vi "Watchdog Extended.vi"(11 "Enable Watchdog":bool=TRUE) -> ()   [LabVIEW 2021]
panel:
  in  "DIOA State":bool
  in  "DIOA Channel":i32=7 min=1 max=50
  in  "Update DIOA":bool=TRUE
  out "Address Found":string
  out "Device Type Found":string
  in  "Reset Device":bool
  in  "Timeout [s]":i32=12 min=1 max=50
  out "Error Message":string="No Error"
  out "error out":errorcluster
  # "Opens the first found U3/U6/UE9 and enables the watchdog to update the state of\na digital output after the specified timeout.  If the DIO is an input, rather than \nan output, this will have no effect.\n\nNote that the UE9 only can also set a 2nd DIO and can set both DAC lines.\n\nNote that it is more common to use \"Config Defaults\" in LJControlPanel to\nconfigure the reset condition of the entire device as desired, then just use the\nwatchdog to reset the device."
  # "DIO must be set to output for this to work.  You can use\n\"U3 Single IO Example.vi\" for that."
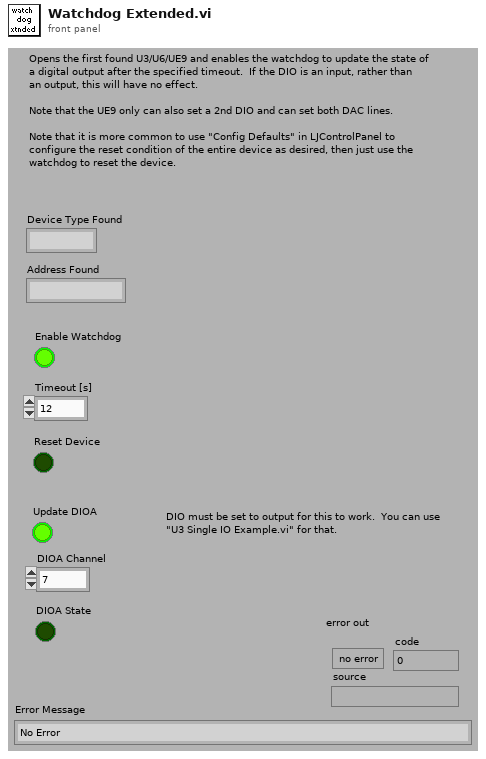
[diagram p1: front panel]
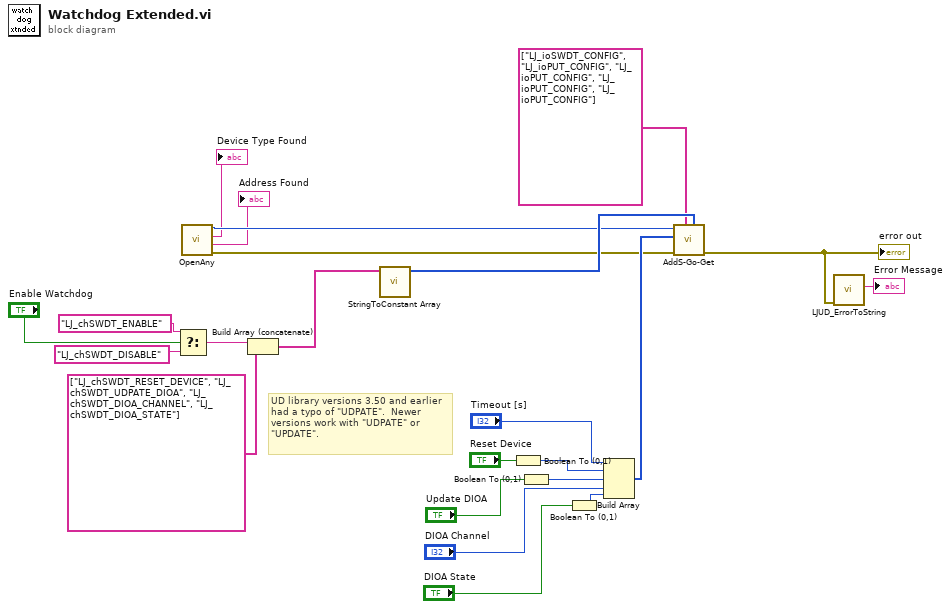
[diagram p0: block diagram]
diagram:
  # "UD library versions 3.50 and earlier\nhad a typo of \"UDPATE\".  Newer\nversions work with \"UDPATE\" or\n\"UPDATE\"."
  n1 = Select(t="LJ_chSWDT_ENABLE" ("IOType"), s="Enable Watchdog", f="LJ_chSWDT_DISABLE" ("IOType")) -> (s? t:f=w6:string)
  n2 = call "OpenAny.vi"() -> ("error out"=w17:errorcluster, "Address Found"=→"Address Found":string, "Device Type Found"=→"Device Type Found":string, "Handle"=w16:i32)  [unwired: 8 in]
  n3 = Build Array (concatenate)(w6, string[] ["LJ_chSWDT_RESET_DEVICE", "LJ_chSWDT_UDPATE_DIOA", "LJ_chSWDT_DIOA_CHANNEL", "LJ_chSWDT_DIOA_STATE"] ("IOTypes")) -> (w4:string[])
  n4 = call "StringToConstant Array.vi"("String Constant Array In"=w4) -> ("I32 Constant Array Out"=w22:i32[])  [unwired: 10 in]
  n5 = Boolean To (0,1)(Boolean="Reset Device") -> (0, 1=w12:i16)
  n6 = Boolean To (0,1)(Boolean="Update DIOA") -> (0, 1=w8:i16)
  n7 = Boolean To (0,1)(Boolean="DIOA State") -> (0, 1=w3:i16)
  n8 = Build Array("Timeout [s]", w12, w8, "DIOA Channel", w3) -> (w18:i32[])
  n9 = call "AddS-Go-Get.vi"("Channels"=w22, "IOTypes"=string[] ["LJ_ioSWDT_CONFIG", "LJ_ioPUT_CONFIG", "LJ_ioPUT_CONFIG", "LJ_ioPUT_CONFIG", "LJ_ioPUT_CONFIG"], "error in"=w17, "Values Write"=w18, "Handle In"=w16) -> ("error out"=w20:errorcluster)  [unwired: 4 in, 2 out]
  "error out" <- w20
  n10 = call "LJUD_ErrorToString.vi"("error in"=w20) -> ("String"=→"Error Message":string)  [unwired: 10 in]
